vi "Hash String with SHA-256.vi"(8 "error In":errorcluster, 11 "String to Encode":string) -> (0 "error Out":errorcluster, 3 "Hash String":string)   [LabVIEW 2018, in "SHA256.lvlib"]
doc: "Calculate a SHA-256 cryptogrpahic hash for a given input string.\n\nImplements the SHA-2 256 encryption algorithm (approximately as described by the wikipedia page pseudocode)."
uses:
  SHA256.lvlib
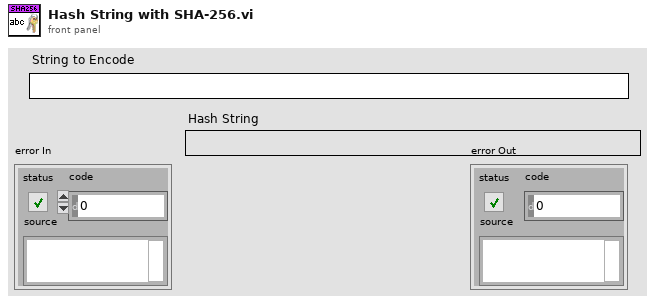
[diagram p1: front panel]
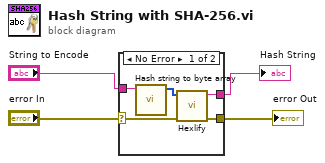
[diagram p0: block diagram]
diagram:
  n1 = case shown="No Error" "error In" {
    selector: "error In" -> [w5 w10]
    tunnel: "String to Encode" -> [w9 _]
    tunnel: [w7 _] -> w3
    tunnel: [w6 w10] -> w2
    frame No Error {
      n2 = call "Hash string to byte array.vi"("String to Encode"=w9) -> ("H Array"=w8:u32[])  [unwired: 10 in]
      n3 = call "Hexlify.vi"("error in (no error)"=w5, "H Array"=w8) -> ("error out"=w6:errorcluster, "String"=w7:string)  [unwired: 8 in]
    }
    frame Error {
    }
  }
  "Hash String" <- w3
  "error Out" <- w2
